vi "PS_Data_Processor.vi"(6 "file path (dialog if empty)":path[](array[path]), 8 "TempCalibOffset":dbl=4.8, 9 "Cell Constant":dbl=0.127, 11 "?":T1=enum."Cond_EIS") -> (0 "time date":string, 1 "Hz":dbl, 2 "TempArray":dbl[](array[numeric]), 3 "Cond (mS)":dbl, 4 "TempCalibOffset 2":dbl=4.8, 5 "Cell Constant 2":dbl=0.33, 7 "Ohms":dbl, 10 "Temp (C)":dbl)   [LabVIEW 2019]
uses:
  5_Controls/PS_CMD_type-def.ctl
  <vilib>/Utility/file.llb/Read Delimited Spreadsheet (string).vi
panel:
  out "lowest phase":dbl
  in  "TempCalibOffset 3":dbl=4.8
  out "all rows":string[][](array[string])
  out "size(s)":i32[](array[numeric])
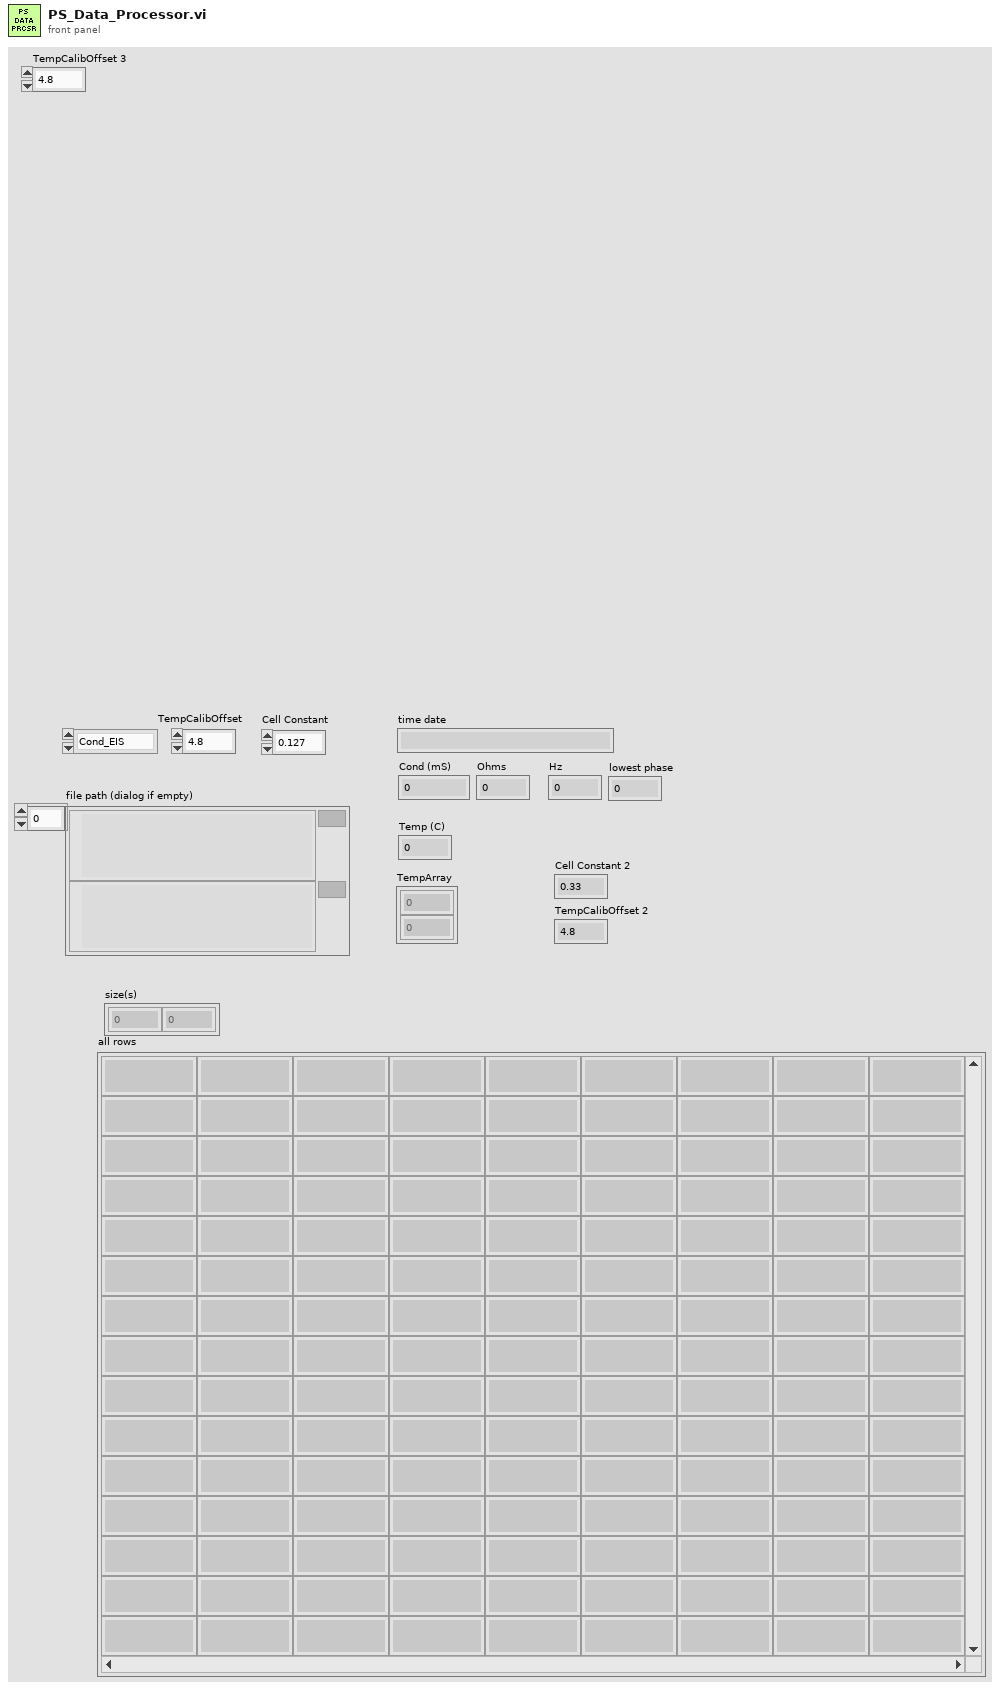
[diagram p1: front panel]
types:
  T1 = typedef "PS_CMD_type-def.ctl" = enum16{"Cond+Temp", "Cond_EIS", "Temp_EIS", "Vwind_MSP", "LongCond", "Cell1_EIS", "Cell2_EIS", "Cell3_EIS"}
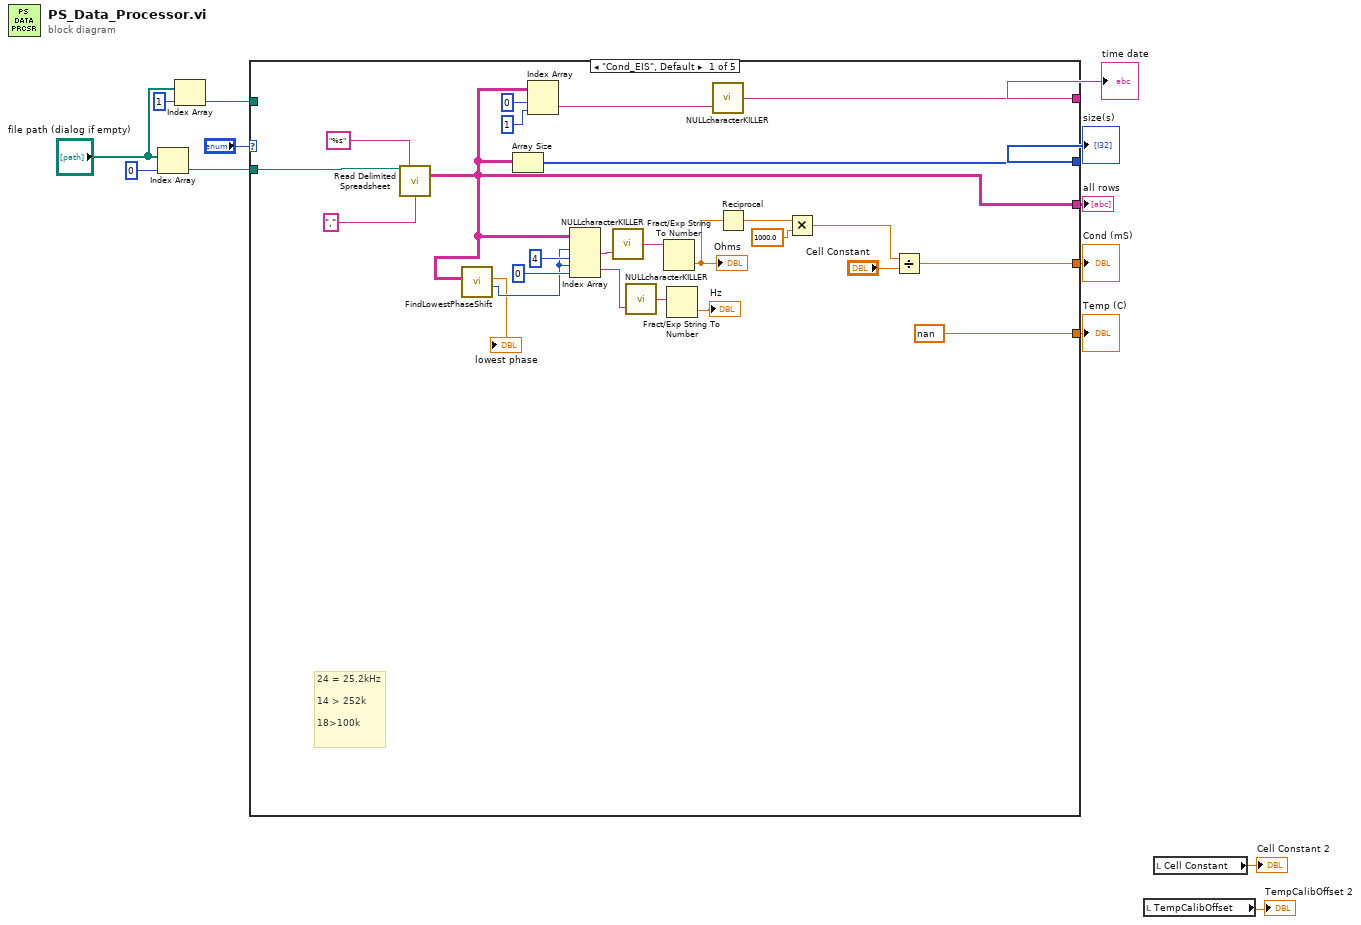
[diagram p0: block diagram]
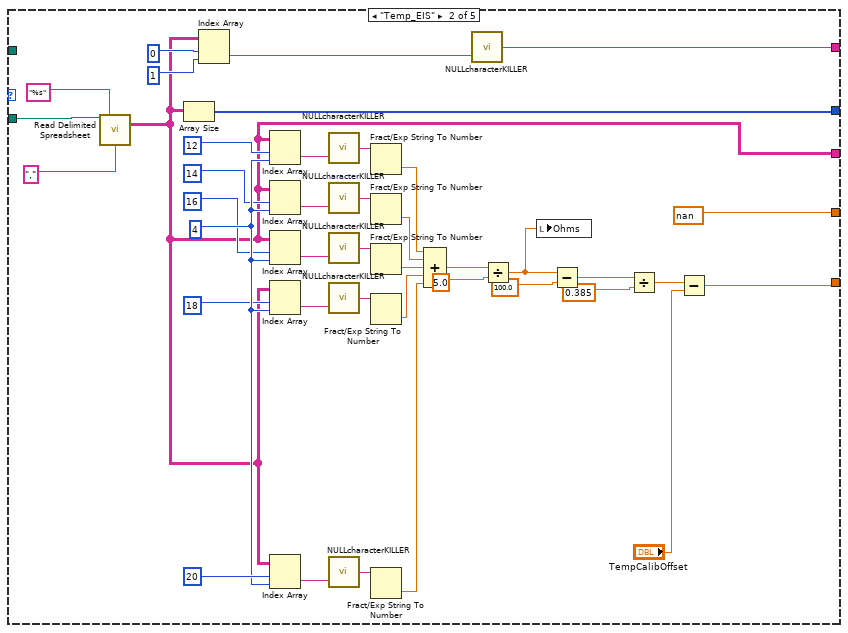
[diagram p2: hidden frame]
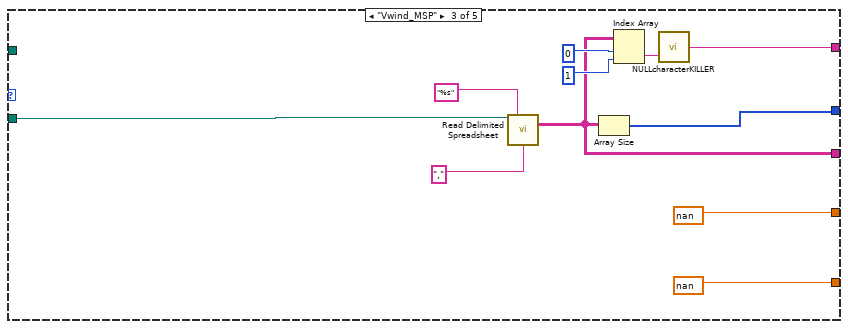
[diagram p3: hidden frame]
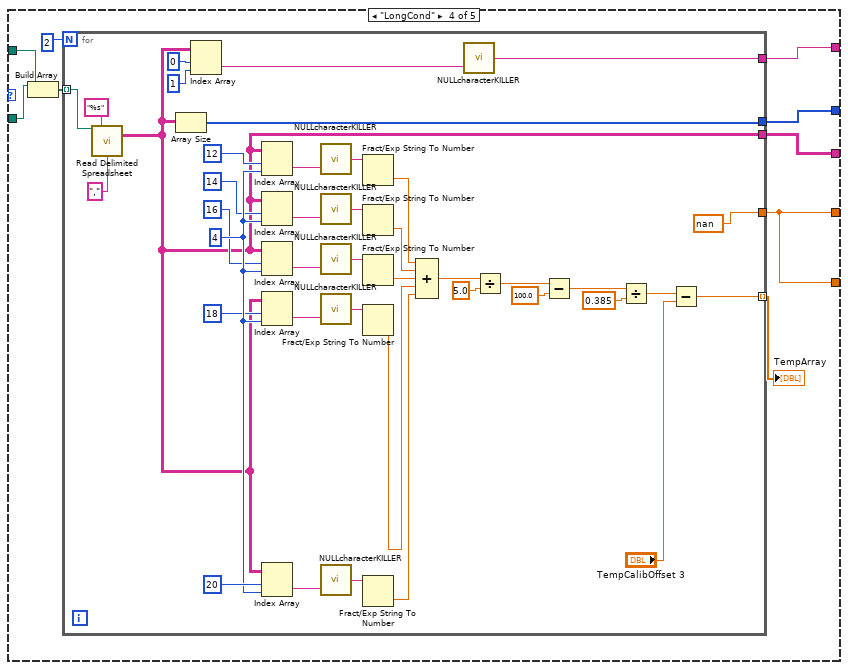
[diagram p4: hidden frame]
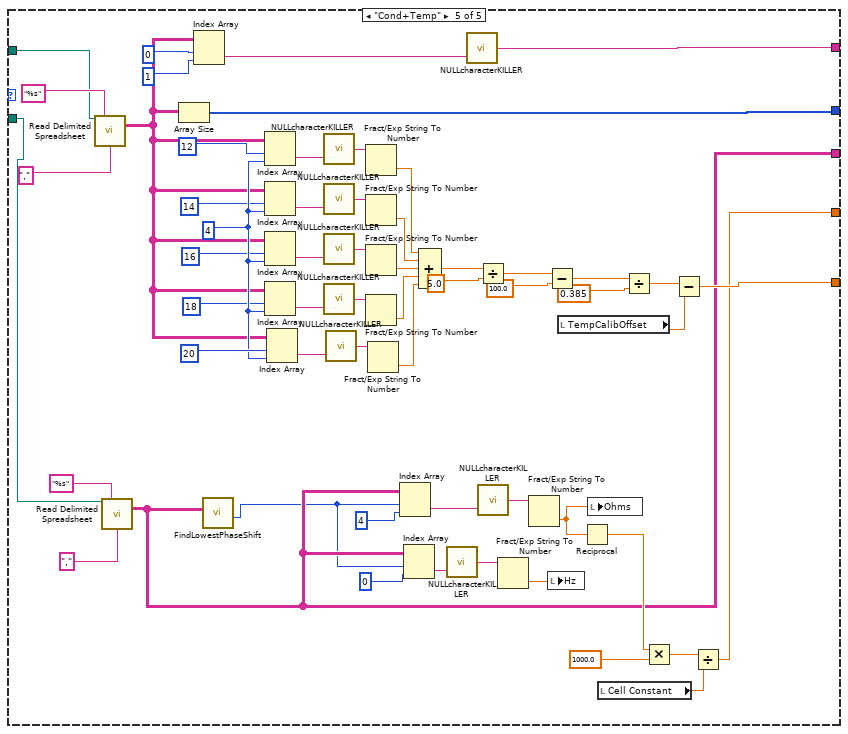
[diagram p5: hidden frame]
diagram:
  n1 = Index Array(array="file path (dialog if empty)", index=0) -> (element=w7:path)
  n2 = Index Array(array="file path (dialog if empty)", index=1) -> (element=w5:path)
  n3 = case shown="\"Cond_EIS\", Default" "?" {
    tunnel: w7 -> [w30 w39 w79 w96 w149]
    tunnel: [w29 nan nan w91 w155] -> w12
    tunnel: [w26 w68 w82 w94 w161] -> w11
    tunnel: [w28 w70 w81 w93 w162] -> w10
    tunnel: [nan w42 nan w91 w160] -> w9
    tunnel: [w16 w46 w80 w92 w142] -> w8
    tunnel: w5 -> [_ _ _ w97 w150]
    frame "Cond_EIS", Default {
      # "24 = 25.2kHz\n\n14 > 252k\n\n18>100k"
      n4 = call-poly <vilib>:"Read Delimited Spreadsheet.vi"("file path (dialog if empty)"=w30, "format (%s)"="%s", "delimiter (\\t)"="," ("delimiter (\\t)")) -> ("all rows"=w16:string[][])  [unwired: 7 in, 5 out]
      n5 = call "FindLowestPhaseShift.vi"("all rows"=w16) -> ("to return"=w15:i32, "lowest phase"=→"lowest phase":dbl)  [unwired: 9 in]
      n6 = Array Size(array=w16) -> (size(s)=w28:i32[])
      n7 = Index Array(array=w16, index (row)=0, index (col)=1 ("disabled index (col)")) -> (element=w27:string)
      n8 = Index Array(array=w16, index (row) #1=w15, index (col) #1=4 ("disabled index (col)"), index (row) #2=w15, index (col) #2=0 ("index (col)")) -> (element #1=w23:string, element #2=w17:string)
      n9 = call "NULLcharacterKILLER.vi"("String"=w23) -> ("string"=w22:string)  [unwired: 1 in]
      n10 = call "NULLcharacterKILLER.vi"("String"=w17) -> ("string"=w20:string)  [unwired: 1 in]
      n11 = Fract/Exp String To Number(string=w22) -> (number=w21:dbl)  [unwired: 3 in, 1 out]
      "Ohms" <- w21
      n12 = Fract/Exp String To Number(string=w20) -> (number=→"Hz":dbl)  [unwired: 3 in, 1 out]
      n13 = call "NULLcharacterKILLER.vi"("String"=w27) -> ("string"=w26:string)  [unwired: 1 in]
      n14 = Reciprocal(x=w21) -> (1/x=w35:dbl)
      n15 = Multiply(x=w35, y=1000.0) -> (x*y=w37:dbl)
      n16 = Divide(x=w37, y="Cell Constant") -> (x/y=w29:dbl)
    }
    frame "Temp_EIS" {
      w67 = 4 ("disabled index (col)")
      n17 = call-poly <vilib>:"Read Delimited Spreadsheet.vi"("file path (dialog if empty)"=w39, "format (%s)"="%s", "delimiter (\\t)"="," ("delimiter (\\t)")) -> ("all rows"=w46:string[][])  [unwired: 7 in, 5 out]
      n18 = Array Size(array=w46) -> (size(s)=w70:i32[])
      n19 = Index Array(array=w46, index (row)=0, index (col)=1 ("disabled index (col)")) -> (element=w69:string)
      n20 = Index Array(array=w46, index (row)=12, index (col)=w67) -> (element=w59:string)
      n21 = Index Array(array=w46, index (row)=14, index (col)=w67) -> (element=w60:string)
      n22 = Index Array(array=w46, index (row)=16, index (col)=w67) -> (element=w61:string)
      n23 = Index Array(array=w46, index (row)=18, index (col)=w67) -> (element=w62:string)
      n24 = Index Array(array=w46, index (row)=20, index (col)=w67) -> (element=w76:string)
      n25 = call "NULLcharacterKILLER.vi"("String"=w59) -> ("string"=w58:string)  [unwired: 1 in]
      n26 = call "NULLcharacterKILLER.vi"("String"=w60) -> ("string"=w57:string)  [unwired: 1 in]
      n27 = call "NULLcharacterKILLER.vi"("String"=w61) -> ("string"=w56:string)  [unwired: 1 in]
      n28 = call "NULLcharacterKILLER.vi"("String"=w62) -> ("string"=w55:string)  [unwired: 1 in]
      n29 = call "NULLcharacterKILLER.vi"("String"=w76) -> ("string"=w77:string)  [unwired: 1 in]
      n30 = Fract/Exp String To Number(string=w58) -> (number=w54:dbl)  [unwired: 3 in, 1 out]
      n31 = Fract/Exp String To Number(string=w57) -> (number=w53:dbl)  [unwired: 3 in, 1 out]
      n32 = Fract/Exp String To Number(string=w56) -> (number=w52:dbl)  [unwired: 3 in, 1 out]
      n33 = Fract/Exp String To Number(string=w55) -> (number=w51:dbl)  [unwired: 3 in, 1 out]
      n34 = Fract/Exp String To Number(string=w77) -> (number=w50:dbl)  [unwired: 3 in, 1 out]
      n35 = Compound Arithmetic op=ADD(w54, w53, w52, w51, w50) -> (w49:dbl)
      n36 = call "NULLcharacterKILLER.vi"("String"=w69) -> ("string"=w68:string)  [unwired: 1 in]
      n37 = Divide(x=w49, y=5.0) -> (x/y=w40:dbl)
      n38 = local write "Ohms"(w40) -> ()
      n39 = Subtract(x=w40, y=100.0) -> (x-y=w44:dbl)
      n40 = Divide(x=w44, y=0.385) -> (x/y=w43:dbl)
      n41 = Subtract(x=w43, y="TempCalibOffset") -> (x-y=w42:dbl)
    }
    frame "Vwind_MSP" {
      n42 = call-poly <vilib>:"Read Delimited Spreadsheet.vi"("file path (dialog if empty)"=w79, "format (%s)"="%s", "delimiter (\\t)"="," ("delimiter (\\t)")) -> ("all rows"=w80:string[][])  [unwired: 7 in, 5 out]
      n43 = Array Size(array=w80) -> (size(s)=w81:i32[])
      n44 = Index Array(array=w80, index (row)=0, index (col)=1 ("disabled index (col)")) -> (element=w87:string)
      n45 = call "NULLcharacterKILLER.vi"("String"=w87) -> ("string"=w82:string)  [unwired: 1 in]
    }
    frame "LongCond" {
      n46 = Build Array(w96, w97) -> (w95:path[])
      n47 = for {
        N: 2 -> [_]
        tunnel: w95 -> [w104] mode=indexing
        tunnel: [w103] -> w94
        tunnel: [w102] -> w93
        tunnel: [w101] -> w92
        tunnel: [nan] -> w91
        tunnel: [w99] -> w90 mode=indexing
        w130 = 4 ("disabled index (col)")
        n48 = call-poly <vilib>:"Read Delimited Spreadsheet.vi"("file path (dialog if empty)"=w104, "format (%s)"="%s", "delimiter (\\t)"="," ("delimiter (\\t)")) -> ("all rows"=w101:string[][])  [unwired: 7 in, 5 out]
        n49 = Array Size(array=w101) -> (size(s)=w102:i32[])
        n50 = Index Array(array=w101, index (row)=0, index (col)=1 ("disabled index (col)")) -> (element=w131:string)
        n51 = Index Array(array=w101, index (row)=12, index (col)=w130) -> (element=w122:string)
        n52 = Index Array(array=w101, index (row)=14, index (col)=w130) -> (element=w123:string)
        n53 = Index Array(array=w101, index (row)=16, index (col)=w130) -> (element=w124:string)
        n54 = Index Array(array=w101, index (row)=18, index (col)=w130) -> (element=w125:string)
        n55 = Index Array(array=w101, index (row)=20, index (col)=w130) -> (element=w137:string)
        n56 = call "NULLcharacterKILLER.vi"("String"=w122) -> ("string"=w121:string)  [unwired: 1 in]
        n57 = call "NULLcharacterKILLER.vi"("String"=w123) -> ("string"=w120:string)  [unwired: 1 in]
        n58 = call "NULLcharacterKILLER.vi"("String"=w124) -> ("string"=w119:string)  [unwired: 1 in]
        n59 = call "NULLcharacterKILLER.vi"("String"=w125) -> ("string"=w118:string)  [unwired: 1 in]
        n60 = call "NULLcharacterKILLER.vi"("String"=w137) -> ("string"=w138:string)  [unwired: 1 in]
        n61 = Fract/Exp String To Number(string=w121) -> (number=w117:dbl)  [unwired: 3 in, 1 out]
        n62 = Fract/Exp String To Number(string=w120) -> (number=w116:dbl)  [unwired: 3 in, 1 out]
        n63 = Fract/Exp String To Number(string=w119) -> (number=w115:dbl)  [unwired: 3 in, 1 out]
        n64 = Fract/Exp String To Number(string=w118) -> (number=w114:dbl)  [unwired: 3 in, 1 out]
        n65 = Fract/Exp String To Number(string=w138) -> (number=w113:dbl)  [unwired: 3 in, 1 out]
        n66 = Compound Arithmetic op=ADD(w117, w116, w115, w114, w113) -> (w112:dbl)
        n67 = call "NULLcharacterKILLER.vi"("String"=w131) -> ("string"=w103:string)  [unwired: 1 in]
        n68 = Divide(x=w112, y=5.0) -> (x/y=w109:dbl)
        n69 = Subtract(x=w109, y=100.0) -> (x-y=w107:dbl)
        n70 = Divide(x=w107, y=0.385) -> (x/y=w106:dbl)
        n71 = Subtract(x=w106, y="TempCalibOffset 3") -> (x-y=w99:dbl)
      }
      "TempArray" <- w90
    }
    frame "Cond+Temp" {
      w187 = 4 ("disabled index (col)")
      n72 = call-poly <vilib>:"Read Delimited Spreadsheet.vi"("file path (dialog if empty)"=w150, "format (%s)"="%s", "delimiter (\\t)"="," ("delimiter (\\t)")) -> ("all rows"=w156:string[][])  [unwired: 7 in, 5 out]
      n73 = call-poly <vilib>:"Read Delimited Spreadsheet.vi"("file path (dialog if empty)"=w149, "format (%s)"="%s", "delimiter (\\t)"="," ("delimiter (\\t)")) -> ("all rows"=w142:string[][])  [unwired: 7 in, 5 out]
      n74 = Array Size(array=w156) -> (size(s)=w162:i32[])
      n75 = Index Array(array=w156, index (row)=0, index (col)=1 ("disabled index (col)")) -> (element=w188:string)
      n76 = call "FindLowestPhaseShift.vi"("all rows"=w142) -> ("to return"=w141:i32)  [unwired: 9 in, 1 out]
      n77 = Index Array(array=w156, index (row)=12, index (col)=w187) -> (element=w179:string)
      n78 = Index Array(array=w156, index (row)=14, index (col)=w187) -> (element=w180:string)
      n79 = Index Array(array=w156, index (row)=16, index (col)=w187) -> (element=w181:string)
      n80 = Index Array(array=w156, index (row)=18, index (col)=w187) -> (element=w182:string)
      n81 = Index Array(array=w156, index (row)=20, index (col)=w187) -> (element=w194:string)
      n82 = call "NULLcharacterKILLER.vi"("String"=w179) -> ("string"=w178:string)  [unwired: 1 in]
      n83 = call "NULLcharacterKILLER.vi"("String"=w180) -> ("string"=w177:string)  [unwired: 1 in]
      n84 = call "NULLcharacterKILLER.vi"("String"=w181) -> ("string"=w176:string)  [unwired: 1 in]
      n85 = call "NULLcharacterKILLER.vi"("String"=w182) -> ("string"=w175:string)  [unwired: 1 in]
      n86 = call "NULLcharacterKILLER.vi"("String"=w194) -> ("string"=w195:string)  [unwired: 1 in]
      n87 = Fract/Exp String To Number(string=w178) -> (number=w174:dbl)  [unwired: 3 in, 1 out]
      n88 = Fract/Exp String To Number(string=w177) -> (number=w173:dbl)  [unwired: 3 in, 1 out]
      n89 = Fract/Exp String To Number(string=w176) -> (number=w172:dbl)  [unwired: 3 in, 1 out]
      n90 = Fract/Exp String To Number(string=w175) -> (number=w171:dbl)  [unwired: 3 in, 1 out]
      n91 = Fract/Exp String To Number(string=w195) -> (number=w170:dbl)  [unwired: 3 in, 1 out]
      n92 = Index Array(array=w142, index (row)=w141, index (col)=4 ("disabled index (col)")) -> (element=w139:string)
      n93 = Index Array(array=w142, index (row)=w141, index (col)=0) -> (element=w140:string)
      n94 = Compound Arithmetic op=ADD(w174, w173, w172, w171, w170) -> (w169:dbl)
      n95 = call "NULLcharacterKILLER.vi"("String"=w140) -> ("string"=w146:string)  [unwired: 1 in]
      n96 = call "NULLcharacterKILLER.vi"("String"=w188) -> ("string"=w161:string)  [unwired: 1 in]
      n97 = Divide(x=w169, y=5.0) -> (x/y=w166:dbl)
      n98 = call "NULLcharacterKILLER.vi"("String"=w139) -> ("string"=w147:string)  [unwired: 1 in]
      n99 = Fract/Exp String To Number(string=w146) -> (number=w143:dbl)  [unwired: 3 in, 1 out]
      n100 = Fract/Exp String To Number(string=w147) -> (number=w144:dbl)  [unwired: 3 in, 1 out]
      n101 = Subtract(x=w166, y=100.0) -> (x-y=w164:dbl)
      n102 = local write "Hz"(w143) -> ()
      n103 = local read "TempCalibOffset"() -> (w153:dbl)
      n104 = Reciprocal(x=w144) -> (1/x=w157:dbl)
      n105 = local write "Ohms"(w144) -> ()
      n106 = local read "Cell Constant"() -> (w154:dbl)
      n107 = Divide(x=w164, y=0.385) -> (x/y=w163:dbl)
      n108 = Multiply(x=w157, y=1000.0) -> (x*y=w159:dbl)
      n109 = Subtract(x=w163, y=w153) -> (x-y=w160:dbl)
      n110 = Divide(x=w159, y=w154) -> (x/y=w155:dbl)
    }
  }
  "Cond (mS)" <- w12
  "time date" <- w11
  "size(s)" <- w10
  "Temp (C)" <- w9
  "all rows" <- w8
  n111 = local read "TempCalibOffset"() -> (→"TempCalibOffset 2":dbl)
  n112 = local read "Cell Constant"() -> (→"Cell Constant 2":dbl)
